vi "IsXYOffsetValid.vi"(7 "Joystick Offset In":T1) -> (1 "IsXYOffsetValid?":bool, 3 "Joystick Offset":T1)   [LabVIEW 2014]
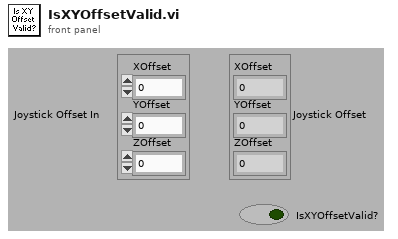
[diagram p1: front panel]
types:
  T1 = cluster{"XOffset":i32, "YOffset":i32, "ZOffset":i32}
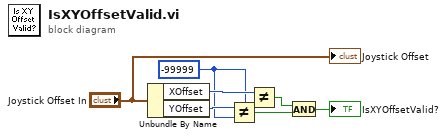
[diagram p0: block diagram]
diagram:
  w4 = -99999 ("XRelPos")
  n1 = Unbundle By Name("Joystick Offset In") -> ("XOffset"=w5:i32, "YOffset"=w6:i32)
  n2 = Not Equal?(x=w6, y=w4) -> (x != y?=w2:bool)
  n3 = Not Equal?(x=w5, y=w4) -> (x != y?=w3:bool)
  n4 = And(x=w3, y=w2) -> (x .and. y?=→"IsXYOffsetValid?":bool)
  "Joystick Offset" <- "Joystick Offset In"
